vi "Introduction.vi"() -> ()   [LabVIEW 2011]
panel:
  out "x > y?":bool
  out "Meter":dbl(knob) scale=0.0..100.0 scale format="%#_3g"
  in  "Knob":dbl(knob) scale=0.0..100.0
  out "Boolean 2":bool
  in  "Boolean":bool
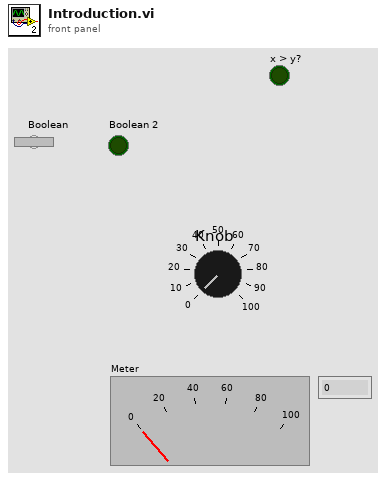
[diagram p1: front panel]
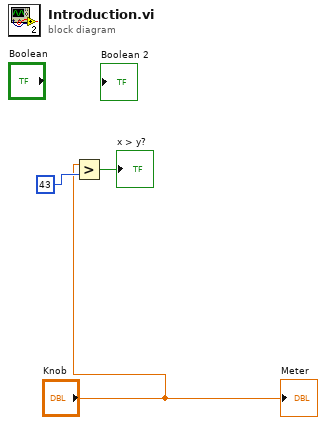
[diagram p0: block diagram]
diagram:
  n1 = Greater?(x="Knob", y=43) -> (0:→"x > y?":bool)
  "Meter" <- "Knob"
